vi "z shm mut data mut.vi"(8 "error in (no error)":errorcluster, 11 "this_":cluster{}) -> (0 "error out":errorcluster, 2 "function return":string, 3 "this_ out":cluster{})   [LabVIEW 2021, in "zenohc.lvlib"]
doc: "unsigned char *z_shm_mut_data_mut(struct z_loaned_shm_mut_t *this_);"
uses:
  zenohc.lvlib
  zenohc.dll
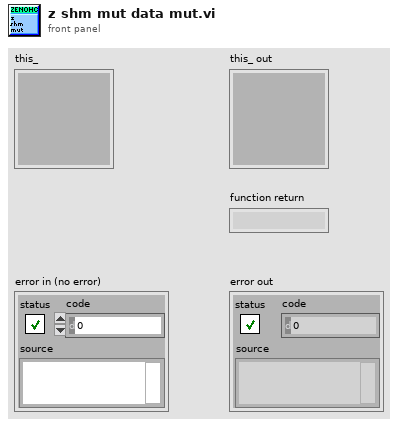
[diagram p1: front panel]
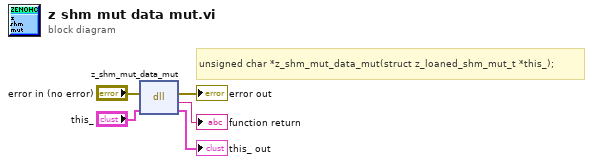
[diagram p0: block diagram]
diagram:
  # "unsigned char *z_shm_mut_data_mut(struct z_loaned_shm_mut_t *this_);"
  n1 = dll-call lib="D:/dev/zenoh_labview/zenohc/zenohc.*" fn="z_shm_mut_data_mut"(error in="error in (no error)", "this_"="this_") -> (error out=→"error out":errorcluster, →"function return":string, "this_"=→"this_ out":cluster{})  [unwired: 2 in, 1 out]
